vi "Ack Fault.vi"(8 "error in (no error)":errorcluster, 11 "controller in":refnum<k24>) -> (0 "error out":errorcluster, 3 "controller out":refnum<k24>)   [LabVIEW 2011]
uses:
  C:/Users/Admin/Desktop/Gantry Code Transfer/source/Code Transfer/Aerotech.A3200.dll
  Aerotech.A3200.dll
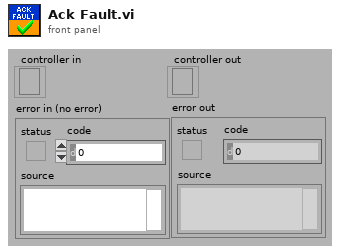
[diagram p1: front panel]
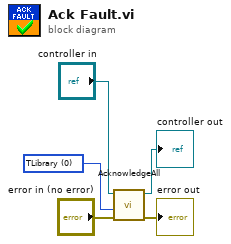
[diagram p0: block diagram]
diagram:
  w1 = 0 items=["TLibrary", "T01", "T02", "T03", "T04", "T05", "T06", "T07", "T08", "T09", "T10", "T11", "T12", "T13", "T14", "T15", "T16", "T17", "T18", "T19", "T20", "T21", "T22", "T23", "T24", "T25", "T26", "T27", "T28", "T29", "T30", "T31"] ("taskId")
  n1 = call "AcknowledgeAll.vi"("error in (no error)"="error in (no error)", "taskId"=w1, "controller in"="controller in") -> ("error out"=→"error out":errorcluster, "controller out"=→"controller out":refnum<k24>)  [unwired: 7 in]
